vi "ReadStatusWord.vi"(8 "error in (no error)":errorcluster, 11 "Motor Base in":refnum<class "Motor Base.lvclass">) -> (0 "error out":errorcluster, 1 "Fault":bool, 2 "Statusword":T1, 3 "Motor Base out":refnum<class "Motor Base.lvclass">)   [LabVIEW 2016, in "Motor Base.lvlib" / "Motor Base.lvclass"]
uses:
  Motor Base.lvclass
  PDS/Statusword.ctl
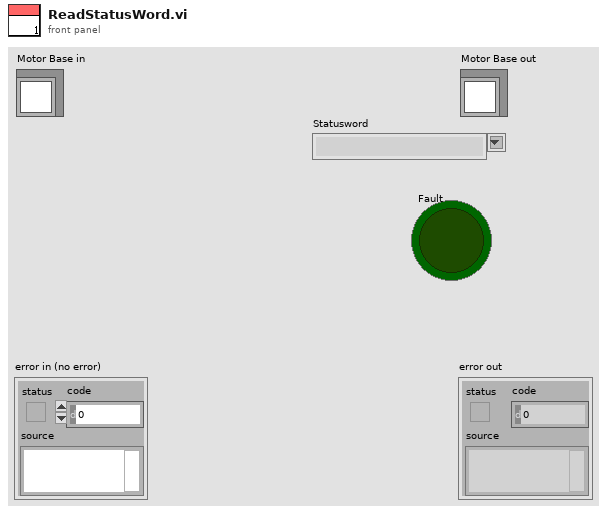
[diagram p1: front panel]
types:
  T1 = typedef "Motor Base.lvlib/Motor Base.lvclass/Statusword.ctl" = string
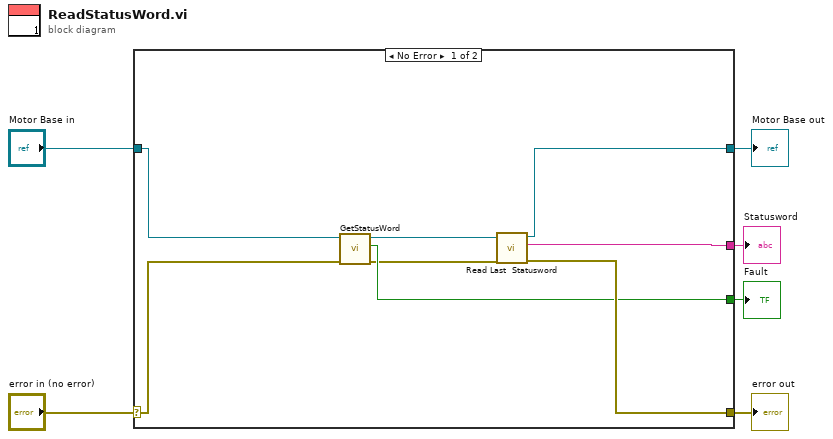
[diagram p0: block diagram]
diagram:
  n1 = case shown="No Error" "error in (no error)" {
    selector: "error in (no error)" -> [w12 w16]
    tunnel: [w11 w16] -> w5
    tunnel: [w13 w15] -> w3
    tunnel: "Motor Base in" -> [w14 w15]
    tunnel: [w10 _] -> w2
    tunnel: [w9 _] -> w1
    frame No Error {
      n2 = call-dynamic "GetStatusWord.vi"("error in (no error)"=w12, "Motor Base in"=w14) -> ("error out"=w7:errorcluster, "Fault"=w10:bool, "Motor Base out"=w8:refnum<class "Motor Base.lvclass">)  [unwired: 7 in]
      n3 = call-dynamic "Read Last  Statusword.vi"("error in (no error)"=w7, "Motor Base in"=w8) -> ("error out"=w11:errorcluster, "Statusword"=w9:T1, "Motor Base out"=w13:refnum<class "Motor Base.lvclass">)  [unwired: 7 in]
    }
    frame Error {
    }
  }
  "error out" <- w5
  "Motor Base out" <- w3
  "Statusword" <- w1
  "Fault" <- w2
